vi "Append.vi"(2 "x":u8[](array[numeric]) format="%02x", 3 "bytestream":refnum<class "Bytestream.lvclass">) -> (1 "bytestream out":refnum<class "Bytestream.lvclass">)   [LabVIEW 2020, in "NI_Bytestream.lvlib" / "Bytestream.lvclass"]
uses:
  <vilib>/Array/Bytestream/Bytestream.lvclass
  <vilib>/Array/Bytestream/Bytestream.lvclass/Bytestream.ctl
  <vilib>/Array/Bytestream/Datum.ctl
  <vilib>/Array/Bytestream/Count Allocated Datums.vi
  <vilib>/Array/Bytestream/Count Datums.vi
  <vilib>/Array/Bytestream/Grow Datum Array.vi
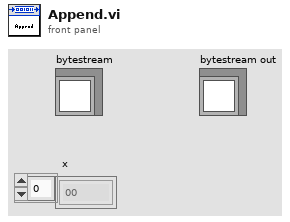
[diagram p1: front panel]
types:
  T1 = typedef "NI_Bytestream.lvlib/Bytestream.lvclass/Datum.ctl" = cluster{"array":u8[], "index":i32}
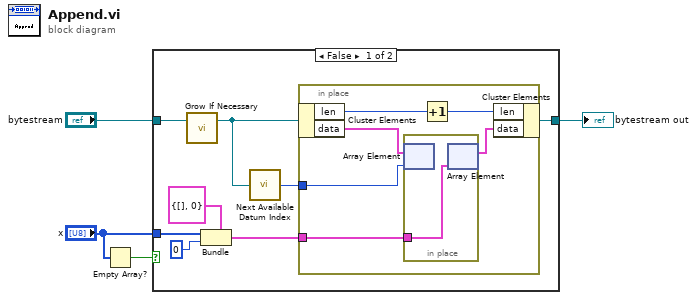
[diagram p0: block diagram]
diagram:
  n1 = Empty Array?(array="x") -> (empty?=w1:bool)
  n2 = case shown="False" w1 {
    tunnel: "bytestream" -> [w8 w20]
    tunnel: [w12 w20] -> w3
    tunnel: "x" -> [w11 _]
    frame False {
      n3 = call <vilib>:"Grow If Necessary.vi"("bytestream in"=w8) -> ("bytestream out"=w7:refnum<class "Bytestream.lvclass">)  [unwired: 2 in]
      n4 = Bundle(cluster=T1 {"array"=[], "index"=0} ("datum"), "array"=w11, "index"=0) -> (w9:T1)
      n5 = call <vilib>:"Next Available Datum Index.vi"("bytestream"=w7) -> ("index"=w6:i32)
      n6 = in-place {
        in-place-border: w9 -> [w16]
        in-place-border: w6 -> [w17]
        n7 = in-place-cluster #1(w7) -> ("len"=w14:i32, "data"=w18:T1[])
        n8 = in-place {
          in-place-border: w16 -> [w19]
          n9 = in-place-array #2(w18, w17) -> ()  [unwired: 1 out]
          n10 = in-place-array #2(w19) -> (w15:T1[])  [unwired: 1 out]
        }
        n11 = Increment(x=w14) -> (x+1=w13:i32)
        n12 = in-place-cluster #1("len"=w13, "data"=w15) -> (w12:refnum<class "Bytestream.lvclass">)
      }
    }
    frame True {
    }
  }
  "bytestream out" <- w3
